vi "main_vi.vi"() -> ()   [LabVIEW 2012]
uses:
  <vilib>/LabVIEW Interface for Arduino/LabVIEW Interface for Arduino.lvlib
  LIFA Ultrasonic Distance LV9/LIFA Ultrasonic Distance.lvlib
  LIFA Ultrasonic Distance LV9/Get Distance/HC-SR04 Get Distance.vi
panel:
  in  "Lines/Points":enum16{"Lines", "Points"}(ring)
  in  "Visible Section":u16(ring)=8
  in  "Grid Color":u32(colorbox)
  in  "Plot Color":u32(colorbox)=16715776
  out "Polar Plot":picture
  out "Angle (Degrees)":u8=15
  in  "Servo 0 Sweep Max Angle":u8=180
  in  "Speed":u8=1
  in  "Signal Pin":u8=9
  in  "Trigger Pin":u8=8
  out "Current distance":dbl
  in  "Stop":bool
  in  "Servo Data Pin":u8=12
  in  "VISA resource":refnum<visa-resource-name>
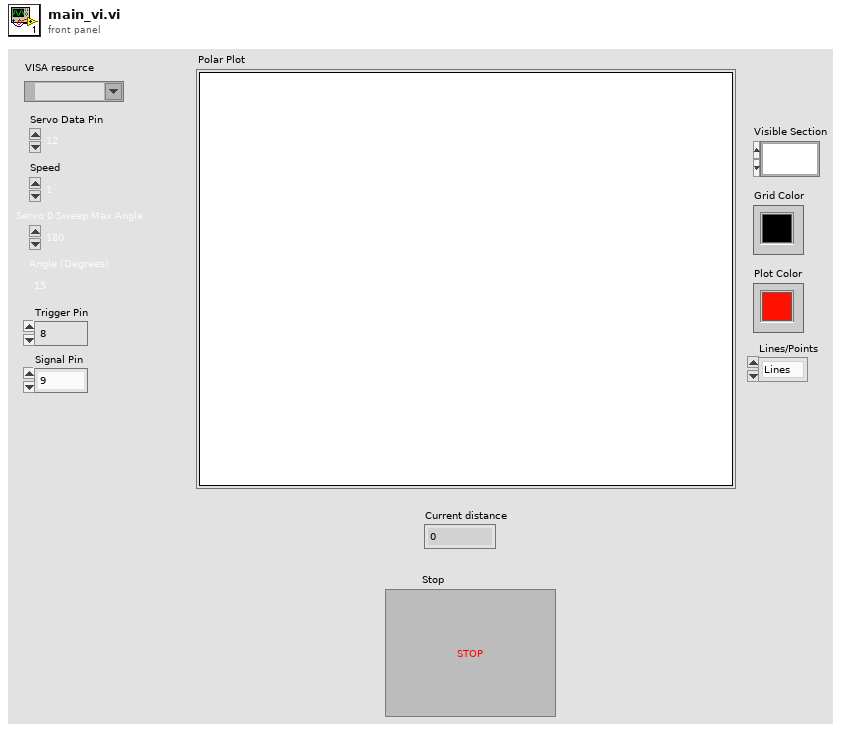
[diagram p1: front panel]
types:
  T1 = cluster{"maximum":dbl, "minimum":dbl, "clip to min":bool, "log?(F)":bool, "grid color":u32, "plot color":u32, "format and precision":cluster{"format":enum8{"Decimal", "Scientific", "Engineering", "Binary", "Octal", "Hex"}, "precision":u8}, "visible section":u16}
  T2 = typedef "LabVIEW Interface for Arduino.lvlib/Arduino Resource.ctl" = cluster{"VISA resource":refnum<visa-resource-name>, "Board Type":T3, "Connection Type":enum8{"USB / Serial"}, "Bytes Per Packet (15)":u8}
  T3 = typedef "LabVIEW Interface for Arduino.lvlib/Board Type.ctl" = enum16{"Uno", "Dimuelanove w/Atmega 328", "Mega 2560"}
  T4 = cluster{"Distance (cm)":dbl, "Angle (Degrees)":u8}
  T5 = typedef "LVBoundsTypeDef.ctl" = cluster{"Width":u32, "Height":u32}
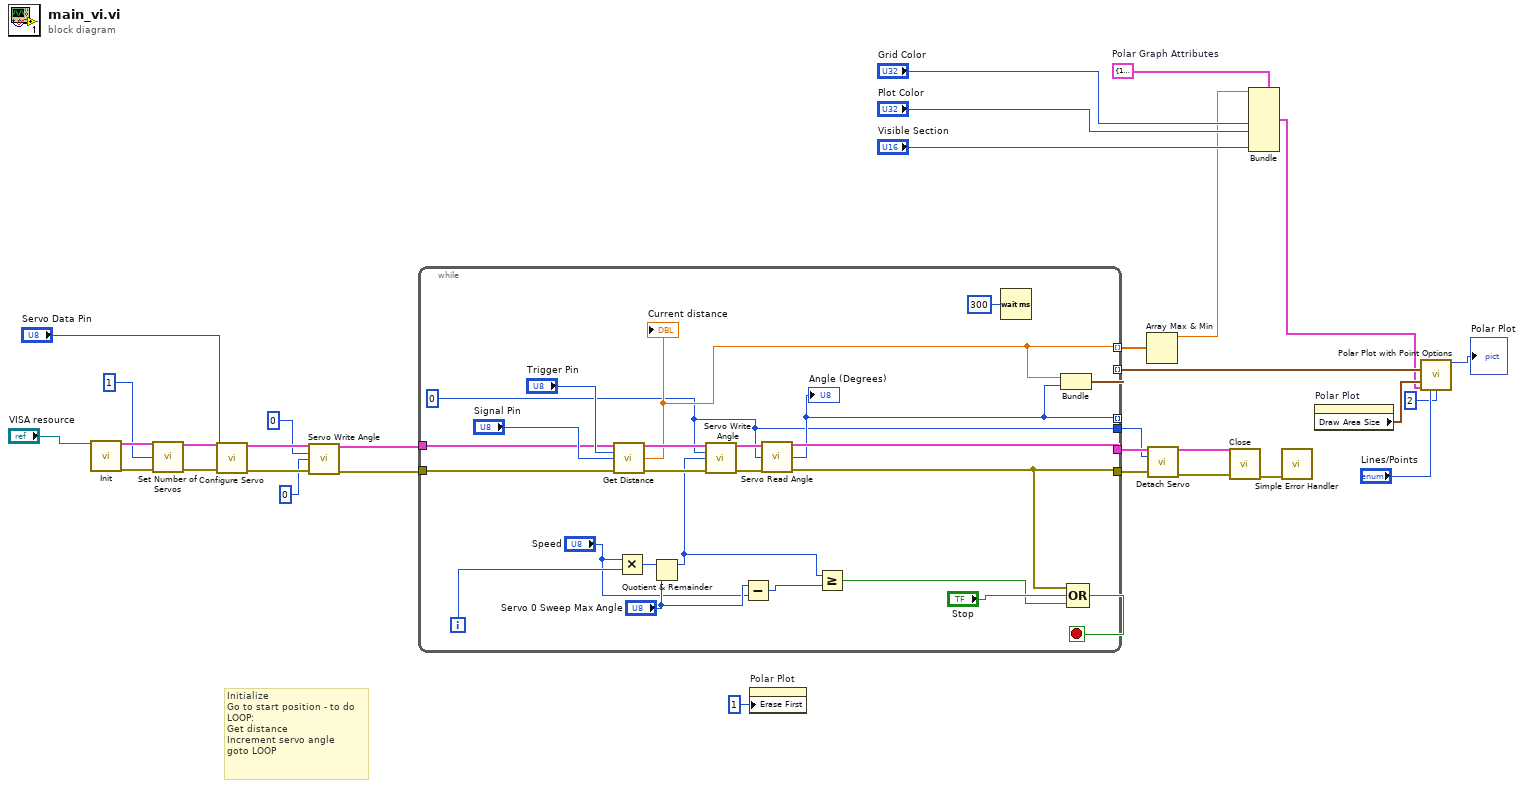
[diagram p0: block diagram]
diagram:
  w18 = T1 {"maximum"=1.0, "minimum"=0.0, "clip to min"=FALSE, "log?(F)"=FALSE, "grid color"=6710886, "plot color"=65280, "format and precision"={"format"=enum."Decimal", "precision"=1}, "visible section"=0}  # Polar Graph Attributes
  # "Initialize\nGo to start position - to do\nLOOP:\nGet distance\nIncrement servo angle\ngoto LOOP"
  n1 = call <vilib>:"Init.vi"("VISA resource"="VISA resource") -> ("Arduino Resource"=w12:T2, "error out"=w11:errorcluster)  [unwired: 17 in]
  n2 = call <vilib>:"Set Number of Servos.vi"("Arduino Resource"=w12, "Number Of Servos (1)"=u8 1, "error in"=w11) -> ("Arduino Resource"=w10:T2, "error out"=w9:errorcluster)  [unwired: 11 in]
  n3 = call <vilib>:"Configure Servo.vi"("Arduino Resource"=w10, "DIO Pin (2)"="Servo Data Pin", "error in"=w9) -> ("Arduino Resource"=w6:T2, "error out"=w5:errorcluster)  [unwired: 11 in]
  n4 = call <vilib>:"Servo Write Angle.vi"("Arduino Resource"=w6, "Servo Number"=u8 0, "Angle (Degrees)"=u8 0, "error in"=w5) -> ("Arduino Resource"=w15:T2, "error out"=w14:errorcluster)  [unwired: 10 in]
  n5 = while {
    tunnel: w15 -> [w35]
    tunnel: w14 -> [w34]
    tunnel: [w47] -> w26
    tunnel: [w45] -> w25
    tunnel: [w43] -> w22 mode=indexing
    tunnel: [w41] -> _ mode=indexing
    tunnel: [w42] -> w28 mode=indexing
    tunnel: [w33] -> w1
    i -> [w50]
    stop <- w44 stop-if-true
    w33 = u8 0 ("Servo Number")
    n6 = call-poly "Get Distance.vi"("Arduino Resource"=w35, "Trigger Pin"="Trigger Pin", "Signal Pin"="Signal Pin", "error in (no error)"=w34) -> ("Arduino Resource"=w55:T2, "Distance (cm)"=w43:dbl, "error out"=w54:errorcluster)  [unwired: 9 in]
    "Current distance" <- w43
    n7 = Multiply(x="Speed", y=w50) -> (x*y=w51:i32)
    n8 = Quotient & Remainder(x=w51, y="Servo 0 Sweep Max Angle") -> (x-y*floor(x/y)=w40:i32)  [unwired: 1 out]
    n9 = call <vilib>:"Servo Write Angle.vi"("Arduino Resource"=w55, "Servo Number"=w33, "Angle (Degrees)"=w40, "error in"=w54) -> ("Arduino Resource"=w49:T2, "error out"=w48:errorcluster)  [unwired: 10 in]
    n10 = Subtract(x="Servo 0 Sweep Max Angle", y="Speed") -> (x-y=w36:u8)
    n11 = call <vilib>:"Servo Read Angle.vi"("Arduino Resource"=w49, "Servo Number"=w33, "error in"=w48) -> ("Arduino Resource"=w47:T2, "Angle (Degrees)"=w41:u8, "error out"=w45:errorcluster)  [unwired: 10 in]
    "Angle (Degrees)" <- w41
    n12 = Greater Or Equal?(x=w40, y=w36) -> (x >= y?=w39:bool)
    n13 = Wait (ms)(milliseconds to wait=u32 300 ("millisecond multiple")) -> ()  [unwired: 1 out]
    n14 = Bundle("Distance (cm)"=w43, "Angle (Degrees)"=w41) -> (w42:T4)  [unwired: 1 in]
    n15 = Compound Arithmetic op=OR(w45, "Stop", w39) -> (w44:bool)
  }
  n16 = property on="Polar Plot" class="Pict"("Erase First"=u8 1) -> ()  [unwired: 2 in, 2 out]
  n17 = Array Max & Min(array=w22) -> (max value=w17:dbl)  [unwired: 3 out]
  n18 = call <vilib>:"Detach Servo.vi"("Arduino Resource"=w26, "Servo Number"=w1, "error in"=w25) -> ("Arduino Resource"=w24:T2, "error out"=w23:errorcluster)  [unwired: 11 in]
  n19 = call <vilib>:"Close.vi"("Arduino Resource"=w24, "error in"=w23) -> ("error out"=w32:errorcluster)  [unwired: 13 in]
  n20 = Bundle(cluster=w18, "maximum"=w17, "grid color"="Grid Color", "plot color"="Plot Color", "visible section"="Visible Section") -> (w16:T1)  [unwired: 4 in]
  n21 = call <vilib>:"Simple Error Handler.vi"("error in (no error)"=w32) -> ()  [unwired: 4 in, 5 out]
  n22 = property on="Polar Plot" class="Pict"() -> ("Draw Area Size"=w30:T5)  [unwired: 2 in, 2 out]
  n23 = call <vilib>:"Polar Plot with Point Options.vi"("data array [mag, phase (deg)]"=w28, "dimensions (w,h)"=w30, "polar attributes"=w16, "Lines/Points"="Lines/Points", "Size"=u16 2) -> ("new picture"=→"Polar Plot":picture)  [unwired: 10 in]
